vi "3-1.vi"() -> ()   [LabVIEW 2022 SP3]
panel:
  out "余弦波":cluster{i32, i32, dbl[]}(graph)
  out "正弦波":dbl[](graph)
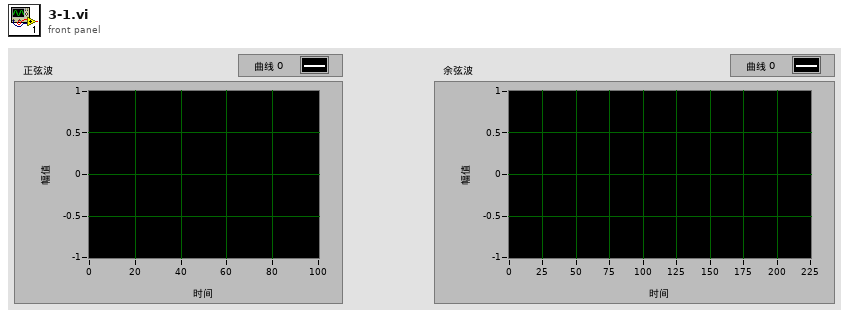
[diagram p1: front panel]
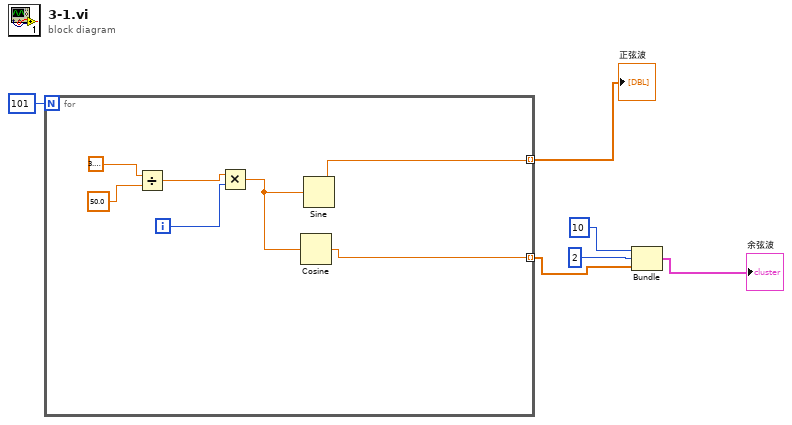
[diagram p0: block diagram]
diagram:
  n1 = for {
    N: 101 -> [_]
    tunnel: [w8] -> w2 mode=indexing
    tunnel: [w7] -> w5 mode=indexing
    i -> [w10]
    n2 = Divide(x=3.141592653589793, y=50.0) -> (x/y=w11:dbl)
    n3 = Multiply(x=w11, y=w10) -> (x*y=w9:dbl)
    n4 = Cosine(x=w9) -> (cos(x)=w8:dbl)
    n5 = Sine(x=w9) -> (sin(x)=w7:dbl)
  }
  "正弦波" <- w5
  n6 = Bundle(10, 2, w2) -> (→"余弦波":cluster{i32, i32, dbl[]})  [unwired: 1 in]
